vi "Write Group Name.vi"(8 "error in (no error)":errorcluster, 10 "Group Name":string, 11 "Mag Lab Result in":refnum<class "Mag Lab Result.lvclass">) -> (0 "error out":errorcluster, 3 "Mag Lab Result out":refnum<class "Mag Lab Result.lvclass">)   [LabVIEW 2015, in "Mag Lab Result.lvclass"]
uses:
  Mag Lab Result.lvclass
  Mag Lab Result.lvclass/Mag Lab Result.ctl
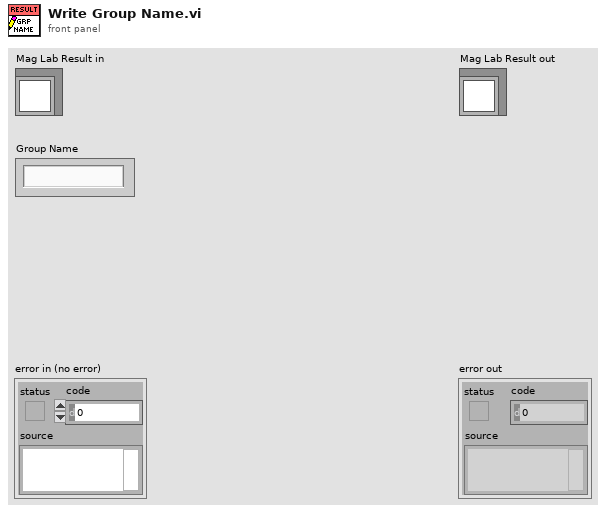
[diagram p1: front panel]
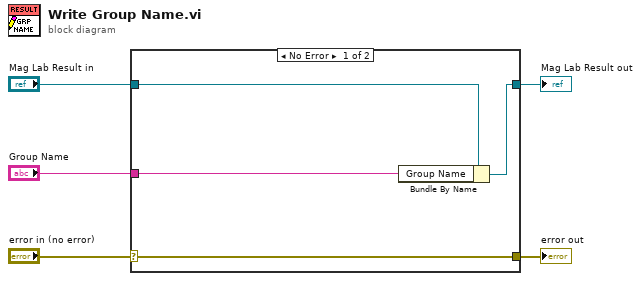
[diagram p0: block diagram]
diagram:
  n1 = case shown="No Error" "error in (no error)" {
    selector: "error in (no error)" -> [w9 w10]
    tunnel: [w9 w10] -> w4
    tunnel: [w7 w11] -> w2
    tunnel: "Mag Lab Result in" -> [w8 w11]
    tunnel: "Group Name" -> [w6 _]
    frame No Error {
      n2 = Bundle By Name(cluster=w8, "Group Name"=w6) -> (w7:refnum<class "Mag Lab Result.lvclass">)
    }
    frame Error {
    }
  }
  "error out" <- w4
  "Mag Lab Result out" <- w2
